vi "Read Data Container.vi"(8 "error in (no error)":errorcluster, 11 "Task_Abstr in":refnum<class "Task_Abstr.lvclass">) -> (0 "error out":errorcluster, 2 "Data Container":refnum<data-value>, 3 "Task_Abstr out":refnum<class "Task_Abstr.lvclass">)   [LabVIEW 2025, in "Task_Abstr.lvlib" / "Task_Abstr.lvclass"]
uses:
  Task_Abstr.lvclass
  Task_Abstr.lvclass/Task_Abstr.ctl
  WaveformData.ctl
  DataContainer.ctl
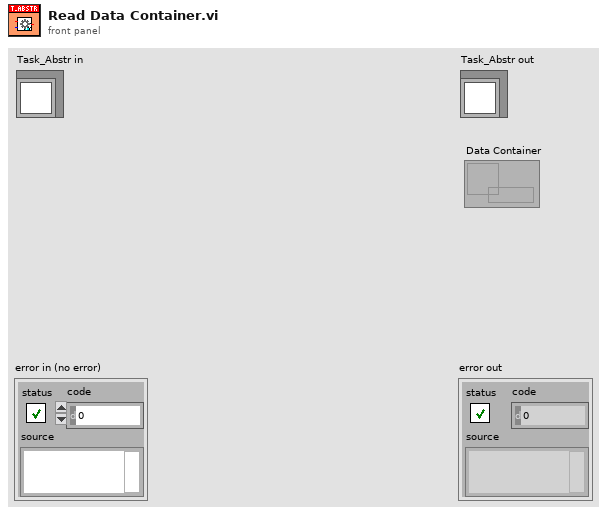
[diagram p1: front panel]
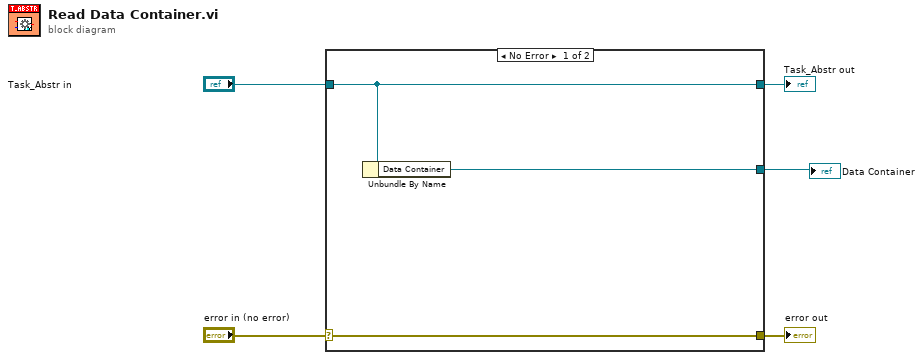
[diagram p0: block diagram]
diagram:
  n1 = case shown="No Error" "error in (no error)" {
    selector: "error in (no error)" -> [w7 w9]
    tunnel: [w7 w9] -> w4
    tunnel: [w8 w10] -> w2
    tunnel: "Task_Abstr in" -> [w8 w10]
    tunnel: [w6 _] -> w1
    frame No Error {
      n2 = Unbundle By Name(w8) -> ("Data Container"=w6:refnum<data-value>)
    }
    frame Error {
    }
  }
  "error out" <- w4
  "Task_Abstr out" <- w2
  "Data Container" <- w1
